vi "Write Not legacy_.vi"(8 "error in (no error)":errorcluster, 10 "Not legacy?":bool, 11 "Motor Configuration in":refnum<class "Motor Configuration.lvclass">) -> (0 "error out":errorcluster, 3 "Motor Configuration out":refnum<class "Motor Configuration.lvclass">)   [LabVIEW 2016, in "Hardware.lvlib" / "Motor.lvlib" / "Motor Configuration.lvclass"]
uses:
  <userlib>/Common Components/Hardware/Motor/Motor Config/Motor Configuration.lvclass
  <userlib>/Common Components/Hardware/Motor/Motor Config/Motor Configuration.lvclass/Motor Configuration.ctl
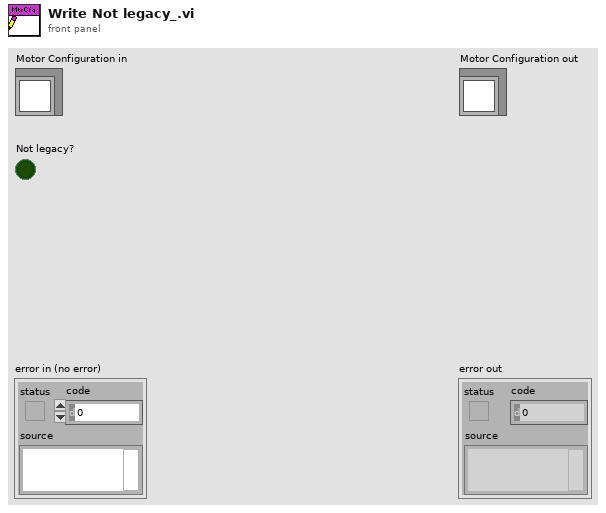
[diagram p1: front panel]
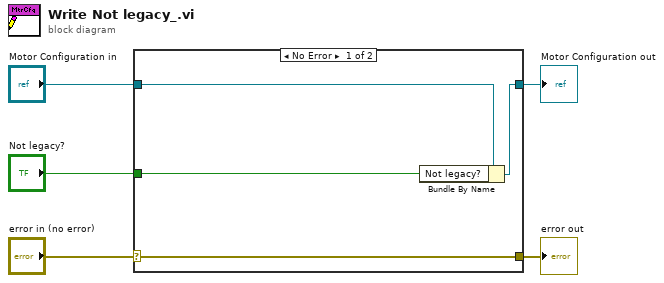
[diagram p0: block diagram]
diagram:
  n1 = case shown="No Error" "error in (no error)" {
    selector: "error in (no error)" -> [w9 w10]
    tunnel: [w9 w10] -> w4
    tunnel: [w7 w11] -> w2
    tunnel: "Motor Configuration in" -> [w8 w11]
    tunnel: "Not legacy?" -> [w6 _]
    frame No Error {
      n2 = Bundle By Name(cluster=w8, "Not legacy?"=w6) -> (w7:refnum<class "Motor Configuration.lvclass">)
    }
    frame Error {
    }
  }
  "error out" <- w4
  "Motor Configuration out" <- w2
